vi "hmi_LM_API_UPD_RESET.vi"(8 "Error in":errorcluster {"code" format="%.0x"}, 11 "canSession":T1) -> (0 "Error out":errorcluster {"code" format="%.0x"}, 3 "canSession":T1)   [LabVIEW 2017]
doc: "Demonstrates how to write and receive CAN frames via the Network Interface on the same port. \n\nTo write and receive frames via the Network Interface:\n- select the CAN Network Interface (i.e. CAN0, CAN1, etc.)\n- select the Baud Rate\n- run the VI\n- press the write button to write frames to the can bus\n\nEnable RTR Button to send a Remote Transmission Request or to simply send an empty Frame to request an Answer Frame from a connected device.\n\nEnable Extended Button to write extended Identifier Format. This is done by setting the 30th bit to enable extended format with the driver."
uses:
  <vilib>/nican/nican.llb/xobjhandle.ctl
  LM_API_UPD.ctl
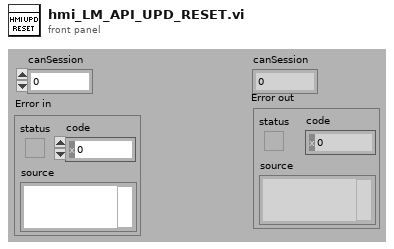
[diagram p1: front panel]
types:
  T1 = typedef "xobjhandle.ctl" = u32
  T2 = typedef "LM_API_UPD.ctl" = u32
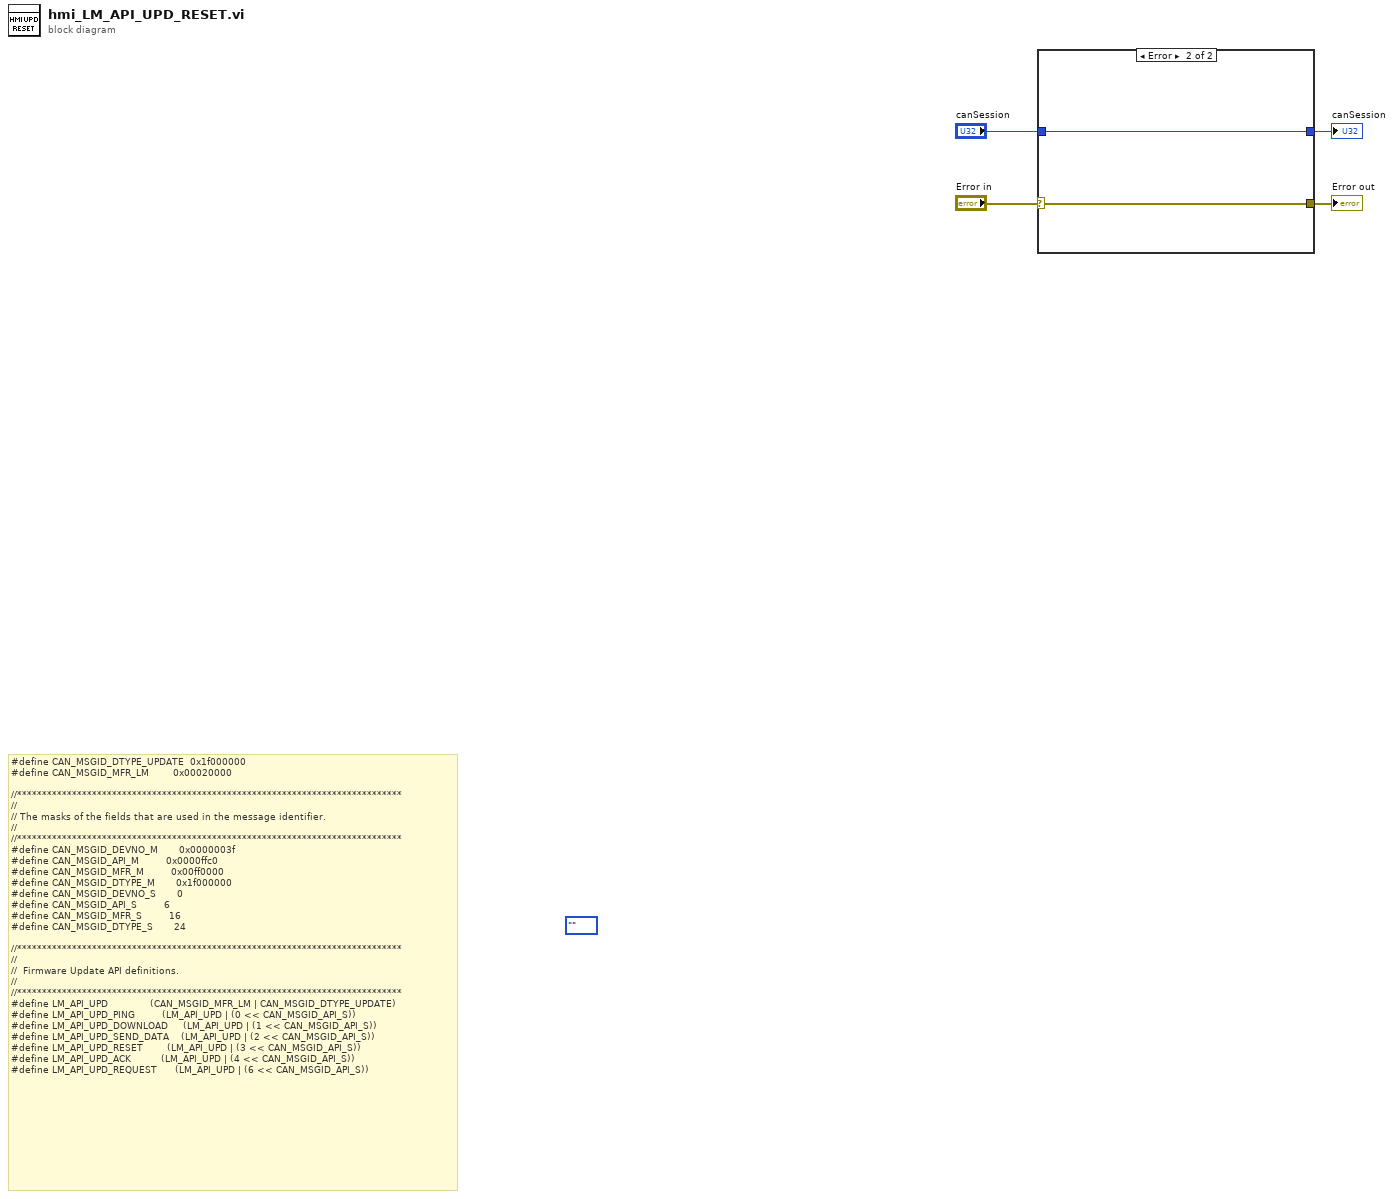
[diagram p0: block diagram]
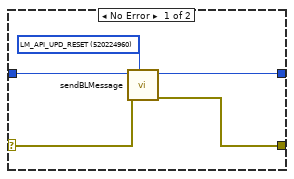
[diagram p2: hidden frame]
diagram:
  (unwired) enum32{""}.""
  # "#define CAN_MSGID_DTYPE_UPDATE  0x1f000000\n#define CAN_MSGID_MFR_LM        0x00020000\n\n//*****************************************************************************\n//\n// The masks of the fields that are used in the message identifier.\n//\n//*****************************************************************************\n#define CAN_MSGID_DEVNO_M       0x0000003f\n#define CAN_MSGID_API_M         0x0000ffc0\n#define CAN_MSGID_MFR_M         0x00ff0000\n#define CAN_MSGID_DTYPE_M       0x1f000000\n#define CAN_MSGID_DEVNO_S       0\n#define CAN_MSGID_API_S         6\n#define CAN_MSGID_MFR_S         16\n#define CAN_MSGID_DTYPE_S       24\n\n//*****************************************************************************\n//\n//  Firmware Update API definitions.\n//\n//*****************************************************************************\n#define LM_API_UPD              (CAN_MSGID_MFR_LM | CAN_MSGID_DTYPE_UPDATE)\n#define LM_API_UPD_PING         (LM_API_UPD | (0 << CAN_MSGID_API_S))\n#define LM_API_UPD_DOWNLOAD     (LM_API_UPD | (1 << CAN_MSGID_API_S))\n#define LM_API_UPD_SEND_DATA    (LM_API_UPD | (2 << CAN_MSGID_API_S))\n#define LM_API_UPD_RESET        (LM_API_UPD | (3 << CAN_MSGID_API_S))\n#define LM_API_UPD_ACK          (LM_API_UPD | (4 << CAN_MSGID_API_S))\n#define LM_API_UPD_REQUEST      (LM_API_UPD | (6 << CAN_MSGID_API_S))"
  n1 = case shown="Error" "Error in" {
    selector: "Error in" -> [w7 w11]
    tunnel: "canSession" -> [w8 w10]
    tunnel: [w5 w10] -> w3
    tunnel: [w6 w11] -> w2
    frame No Error {
      w9 = T2 520224960 items=["LM_API_UPD_PING"=520224768, "LM_API_UPD_DOWNLOAD"=520224780, "LM_API_UPD_SEND_DATA"=520224792, "LM_API_UPD_RESET"=520224960, "LM_API_UPD_ACK"=520224864, "LM_API_UPD_REQUEST"=520227516]
      n2 = call "sendBLMessage.vi"("blMessage"=w9, "Error in"=w7, "ObjHandle in"=w8) -> ("Error out"=w6:errorcluster, "ObjHandle out"=w5:T1)  [unwired: 7 in]
    }
    frame Error {
    }
  }
  "canSession" <- w3
  "Error out" <- w2
